vi "ingest_containerized.vi"(4 "tag":string, 6 "extractorRid":string, 8 "error in":errorcluster, 9 "Target":refnum<class "target.lvclass">, 10 "sources":refnum<class "source.lvclass">[](array[class]), 11 "Nominal Client in":refnum<class "Nominal Client.lvclass">) -> (0 "error out":errorcluster, 1 "datasetRid":string, 2 "datasetFileId":string, 3 "Nominal Client out":refnum<class "Nominal Client.lvclass">)   [LabVIEW 2020, in "Nominal Client.lvclass"]
doc: "Triggers an ingest job, allowing either creating a new dataset or uploading to an existing one. This endpoint is meant to supersede all other ingestion endpoints as their functionality gets migrated to this one."
uses:
  Nominal Client.lvclass
  datasources/target/target.lvclass
  datasources/source/source.lvclass
  Nominal Client.lvclass/Nominal Client.ctl
  datasources/target/target.lvclass/target.ctl
  51a8208b-abcd-4ca2-9510-7220a654322d.vi
  6c2804b0-e365-4e4a-89a7-22827fb1f174.vi
  d08c04c5-7678-4b16-ba2b-d4dd41cd1ace.vi
  datasources/target/workspace.set.vi
  <vilib>/JDP Science/JSONtext/Variant to JSON Text.vi
  <vilib>/JDP Science/JSONtext/support/Format JSON Array Text.vi
  <vilib>/JDP Science/JSONtext/support/Format JSON Object.vi
  <vilib>/JDP Science/JSONtext/JSON text to Variant.vi
  <vilib>/JDP Science/JSONtext/LVClass Serializer/JSONtext LVClass Serializer.lvclass
  <vilib>/JDP Science/JSONtext/JSONtext.lvlib
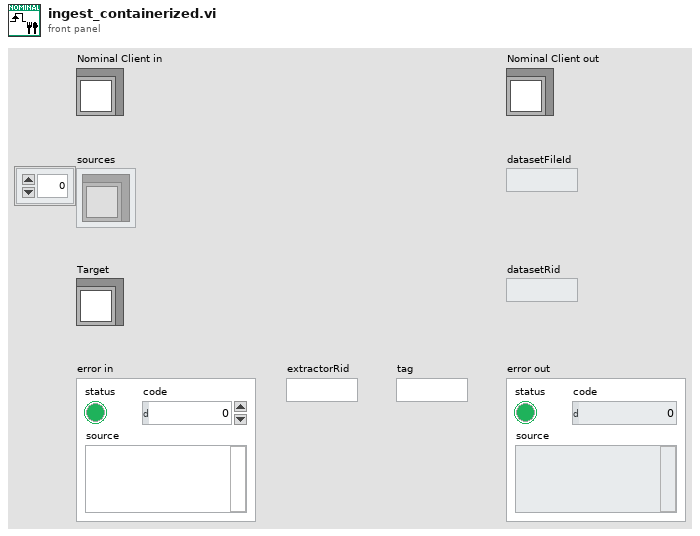
[diagram p1: front panel]
types:
  T1 = cluster{"type":string, "dataset":cluster{"datasetFileId":string, "datasetRid":string}}
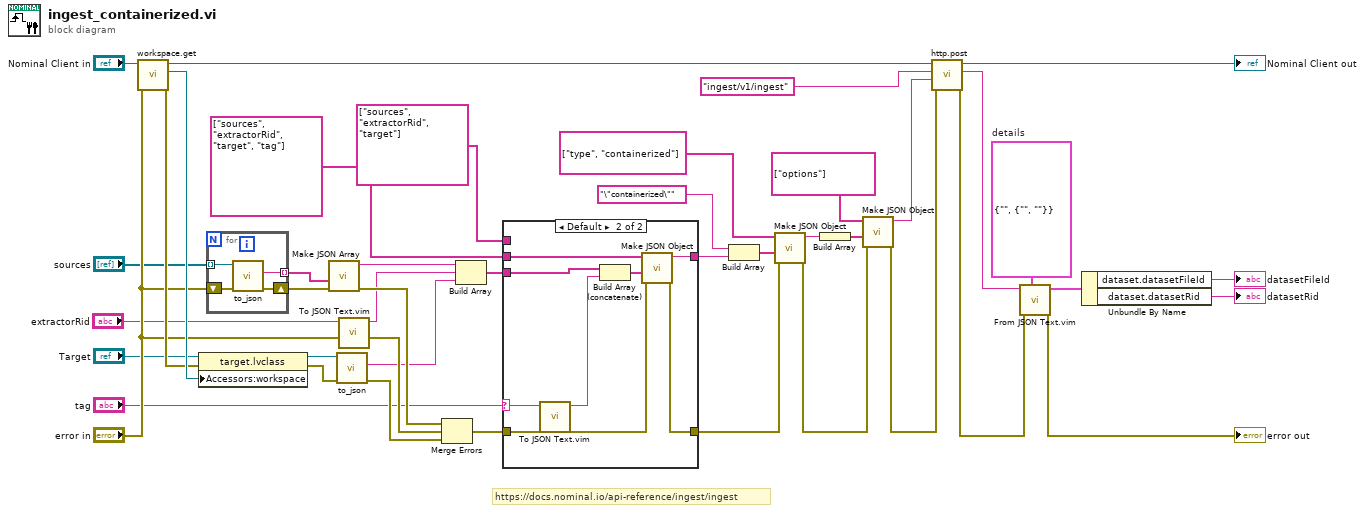
[diagram p0: block diagram]
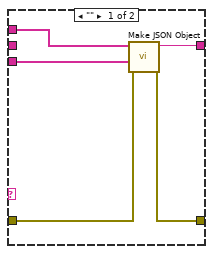
[diagram p2: hidden frame]
diagram:
  w13 = T1 {"type"="", "dataset"={"datasetFileId"="", "datasetRid"=""}}  # details
  # "https://docs.nominal.io/api-reference/ingest/ingest"
  n1 = call "workspace.get.vi"("error in"="error in", "Nominal Client in"="Nominal Client in") -> ("error out"=w35:errorcluster, "workspace"=w37:refnum<class "workspace.lvclass">, "Nominal Client out"=w38:refnum<class "Nominal Client.lvclass">)  [unwired: 7 in]
  n2 = property class="target.lvclass"(reference="Target", error in=w35, "Accessors:workspace"=w37) -> (reference out=w40:refnum<class "target.lvclass">, error out=w41:errorcluster)
  n3 = for {
    tunnel: "sources" -> [w46] mode=indexing
    tunnel: [w45] -> w32 mode=indexing
    shift-right: [w47] -> w30
    shift-left: "error in" -> [w44]
    n4 = call-dynamic "to_json.vi"("error in"=w44, "source in"=w46) -> ("error out"=w47:errorcluster, "json"=w45:string)  [unwired: 6 in, 2 out]
  }
  n5 = call <vilib>:"Make JSON Array.vi"("error in (no error)"=w30, "JSON Elements"=w32) -> ("error out"=w29:errorcluster, "<JSON>"=w31:string)  [unwired: 8 in]
  n6 = call-dynamic "to_json.vi"("error in"=w41, "target in"=w40) -> ("error out"=w27:errorcluster, "json"=w24:string)  [unwired: 6 in, 2 out]
  n7 = call "To JSON Text.vim"("error in (no error)"="error in", "Anything"="extractorRid") -> ("error out"=w26:errorcluster, "<JSON>"=w25:string)  [unwired: 8 in]
  n8 = Merge Errors(w29, w26, w27) -> (w36:errorcluster)
  n9 = Build Array(w31, w25, w24) -> (w33:string[])
  n10 = case shown="Default" "tag" {
    selector: "tag" -> [_ w53]
    tunnel: w36 -> [w49 w58]
    tunnel: string[] ["sources", "extractorRid", "target", "tag"] -> [_ w61]
    tunnel: w33 -> [w52 w56]
    tunnel: [w51 w60] -> w17
    tunnel: [w48 w59] -> w14
    tunnel: string[] ["sources", "extractorRid", "target"] -> [w50 _]
    frame "" {
      n11 = call <vilib>:"Make JSON Object.vi"("error in (no error)"=w49, "JSON Items"=w52, "Item Names"=w50) -> ("error out"=w48:errorcluster, "<JSON>"=w51:string)  [unwired: 7 in]
    }
    frame Default {
      n12 = call "To JSON Text.vim"("error in (no error)"=w58, "Anything"=w53) -> ("error out"=w57:errorcluster, "<JSON>"=w54:string)  [unwired: 8 in]
      n13 = Build Array (concatenate)(w56, w54) -> (w55:string[])
      n14 = call <vilib>:"Make JSON Object.vi"("error in (no error)"=w57, "JSON Items"=w55, "Item Names"=w61) -> ("error out"=w59:errorcluster, "<JSON>"=w60:string)  [unwired: 7 in]
    }
  }
  n15 = Build Array("\"containerized\"" ("JSON"), w17) -> (w15:string[])
  n16 = call <vilib>:"Make JSON Object.vi"("error in (no error)"=w14, "JSON Items"=w15, "Item Names"=string[] ["type", "containerized"] ("JSON")) -> ("error out"=w2:errorcluster, "<JSON>"=w6:string)  [unwired: 7 in]
  n17 = Build Array(w6) -> (w5:string[])
  n18 = call <vilib>:"Make JSON Object.vi"("error in (no error)"=w2, "JSON Items"=w5, "Item Names"=string[] ["options"] ("JSON")) -> ("error out"=w1:errorcluster, "<JSON>"=w4:string)  [unwired: 7 in]
  n19 = call "http.post.vi"("error in"=w1, "Request body"=w4, "Path"="ingest/v1/ingest", "Nominal Client in"=w38) -> ("error out"=w8:errorcluster, "Response"=w9:string, "Nominal Client out"=→"Nominal Client out":refnum<class "Nominal Client.lvclass">)  [unwired: 4 in, 1 out]
  n20 = call "From JSON Text.vim"("Data Type and Default Value"=w13, "error in (no error)"=w8, "JSON"=w9) -> ("error out"=→"error out":errorcluster, "Data out"=w12:T1)  [unwired: 7 in]
  n21 = Unbundle By Name(w12) -> ("dataset.datasetFileId"=→"datasetFileId":string, "dataset.datasetRid"=→"datasetRid":string)
